vi "CCD-2D-RTmode.vi"() -> ()   [LabVIEW 2021]
uses:
  Globals and TypeDefs/gDetector.vi
panel:
  out "Processing":u32
  out "Read":u32
  out "RQS":u32
  out "Start":u32
  in  "stop":bool
  out "Plot":i32[](graph)
  in  "Shutter Enabled":bool=TRUE
  out "\"ST\" status":bool[](array[boolean])
  in  "Exposuretime (s)":dbl=0.5 format="%.2f"
  in  "CCD GPIB Address":u16=1
  out "error out":errorcluster
  out "The Data":i32[][](array[numeric])=[[1198, 1190, 1193, 1194, 1189, 1188, 1196, 1190, 1202, 1191, 1193, 1192, 1199, 1189, 1194, 1189, 1197, 1191, 1187, 1192, 1195, 1189, 1195, 1191, 1199, 1194, 1192, 1191, 1193, 1197, 1193, 1193, 1194, 1200, 1191, 1190, 1187, 1195, 1189, 1188, 1191, 1194, 1187, 1192, 1198, 1193, 1190, 1192, 1190, 1193, 1191, 1190, 1191, 1189, 1192, 1194, 1190, 1193, 1193, 1191, 1194, 1182, 1190, 1188, 1199, 1192, 1196, 1195, 1186, 1189, 1188, 1185, 1194, 1187, 1193, 1194, 1190, 1189, 1189, 1187, 1196, 1195, 1191, 1197, 1192, 1200, 1187, 1194, 1189, 1193, 1195, 1196, 1186, 1192, 1190, 1194, 1194, 1190, 1191, 1193, 1197, 1197, 1185, 1199, 1190, 1195, 1196, 1184, 1193, 1193, 1193, 1191, 1189, 1190, 1199, 1193, 1191, 1194, 1191, 1192, 1186, 1190, 1194, 1189, 1194, 1190, 1191, 1192, 1192, 1196, 1192, 1192, 1189, 1193, 1198, 1186, 1191, 1193, 1187, 1194, 1190, 1190, 1191, 1189, 1194, 1195, 1189, 1192, 1185, 1193, 1192, 1192, 1189, 1191, 1191, 1190, 1196, 1194, 1193, 1191, 1189, 1191, 1196, 1192, 1192, 1189, 1196, 1191, 1193, 1192, 1188, 1190, 1194, 1192, 1185, 1191, 1194, 1191, 1189, 1195, 1192, 1196, 1190, 1193, 1191, 1189, 1194, 1195, 1191, 1187, 1190, 1196, 1196, 1192, 1197, 1191, 1189, 1192, 1192, 1200, 1192, 1193, 1190, 1192, 1187, 1198, 1186, 1196, 1201, 1199, 1200, 1191, 1196, 1200, 1192, 1191, 1193, 1185, 1192, 1194, 1186, 1190, 1188, 1189, 1201, 1197, 1191, 1194, 1193, 1194, 1195, 1198, 1200, 1192, 1192, 1193, 1193, 1195, 1187, 1193, 1192, 1187, 1189, 1186, 1191, 1197, 1191, 1200, 1194, 1192, 1187, 1196, 1191, 1191, 1196, 1187, 1190, 1193, 1189, 1193, 1190, 1188, 1188, 1190, 1197, 1188, 1191, 1195, 1188, 1191, 1188, 1194, 1193, 1187, 1200, 1192, 1197, 1190, 1196, 1200, 1191, 1189, 1193, 1189, 1186, 1196, 1185, 1198, 1195, 1186, 1191, 1197, 1191, 1193, 1195, 1193, 1191, 1198, 1189, 1183, 1200, 1197, 1192, 1192, 1192, 1196, 1191, 1190, 1194, 1188, 1198, 1193, 1195, 1190, 1187, 1192, 1191, 1195, 1188, 1190, 1191, 1187, 1189, 1185, 1189, 1196, 1198, 1191, 1190, 1196, 1197, 1193, 1187, 1186, 1195, 1191, 1193, 1192, 1196, 1190, 1192, 1192, 1192, 1190, 1195, 1192, 1191, 1193, 1197, 1184, 1190, 1188, 1192, 1194, 1190, 1193, 1195, 1195, 1194, 1189, 1193, 1191, 1194, 1186, 1189, 1192, 1191, 1182, 1190, 1197, 1194, 1188, 1193, 1191, 1186, 1194, 1197, 1193, 1191, 1187, 1194, 1194, 1191, 1189, 1195, 1194, 1189, 1196, 1187, 1186, 1192, 1194, 1196, 1191, 1193, 1191, 1188, 1190, 1199, 1198, 1196, 1196, 1190, 1194, 1191, 1194, 1187, 1195, 1190, 1194, 1196, 1194, 1189, 1193, 1189, 1194, 1189, 1195, 1192, 1194, 1193, 1191, 1197, 1187, 1189, 1189, 1188, 1197, 1192, 1189, 1193, 1194, 1183, 1202, 1187, 1192, 1184, 1188, 1186, 1193, 1189, 1195, 1189, 1193, 1197, 1189, 1194, 1191, 1194, 1192, 1191, 1191, 1196, 1194, 1190, 1193, 1192, 1195, 1197, 1198, 1193, 1202, 1196, 1194, 1194, 1190, 1193, 1190, 1195, 1192, 1187, 1194, 1197, 1190, 1194, 1189, 1198, 1192, 1191, 1192, 1192, 1191, 1191, 1193, 1191, 1191, 1198, 1186, 1192, 1185, 1185, 1188, 1194, 1196, 1194, 1195, 1190, 1194, 1191, 1190, 1195, 1191, 1191, 1195, 1192, 1194, 1201, 1187, 1191, 1195, 1187, 1192, 1192, 1193, 1200, 1188, 1189, 1189, 1197, 1189, 1188, 1197, 1195, 1191, 1189, 1190, 1195, 1189, 1191, 1194, 1186, 1192, 1190, 1191, 1188, 1195, 1192, 1191, 1191, 1199, 1190, 1190, 1190, 1192, 1187, 1193, 1197, 1197, 1186, 1193, 1189, 1192, 1197, 1184, 1187, 1188, 1192, 1192, 1192, 1189, 1192, 1190, 1194, 1191, 1186, 1196, 1194, 1189, 1193, 1191, 1186, 1189, 1193, 1195, 1196, 1197, 1199, 1194, 1190, 1193, 1194, 1190, 1198, 1196, 1194, 1195, 1194, 1184, 1188, 1195, 1197, 1190, 1194, 1190, 1191, 1195, 1198, 1188, 1193, 1194, 1195, 1198, 1195, 1191, 1197, 1192, 1198, 1190, 1196, 1191, 1194, 1188, 1189, 1198, 1192, 1198, 1195, 1185, 1191, 1193, 1192, 1197, 1195, 1195, 1195, 1193, 1190, 1190, 1190, 1198, 1195, 1191, 1194, 1190, 1190, 1194, 1194, 1195, 1192, 1190, 1194, 1195, 1192, 1192, 1194, 1189, 1192, 1193, 1188, 1194, 1195, 1196, 1193, 1192, 1201, 1191, 1198, 1197, 1191, 1192, 1191, 1194, 1193, 1188, 1192, 1189, 1183, 1189, 1190, 1192, 1189, 1196, 1193, 1197, 1185, 1193, 1189, 1191, 1196, 1195, 1193, 1193, 1191, 1189, 1193, 1192, 1192, 1192, 1190, 1191, 1193, 1193, 1197, 1195, 1189, 1193, 1188, 1194, 1197, 1194, 1195, 1196, 1190, 1194, 1188, 1197, 1195, 1191, 1195, 1192, 1194, 1188, 1190, 1197, 1197, 1191, 1187, 1197, 1191, 1193, 1188, 1191, 1194, 1193, 1195, 1192, 1195, 1189, 1193, 1193, 1195, 1190, 1192, 1196, 1188, 1187, 1193, 1192, 1192, 1194, 1185, 1199, 1190, 1193, 1191, 1198, 1189, 1190, 1191, 1190, 1193, 1195, 1186, 1190, 1193, 1191, 1189, 1197, 1193, 1198, 1190, 1192, 1193, 1191, 1196, 1193, 1196, 1190, 1190, 1198, 1192, 1199, 1198, 1190, 1191, 1191, 1196, 1190, 1196, 1195, 1191, 1196, 1195, 1193, 1190, 1190, 1195, 1193, 1187, 1197, 1185, 1191, 1189, 1191, 1193, 1192, 1188, 1196, 1193, 1191, 1193, 1193, 1190, 1192, 1192, 1192, 1195, 1191, 1195, 1189, 1189, 1191, 1191, 1185, 1192, 1191, 1193, 1201, 1199, 1197, 1206, 1201, 1207, 1200, 1198, 1195, 1188, 1194, 1186, 1190, 1197, 1188, 1193, 1196, 1193, 1192, 1192, 1188, 1196, 1186, 1193, 1194, 1188, 1190, 1190, 1192, 1190, 1191, 1191, 1200, 1192, 1199, 1193, 1190, 1190, 1199, 1187, 1193, 1190, 1188, 1194, 1194, 1196, 1194, 1195, 1190, 1187, 1187, 1196, 1193, 1199, 1190, 1193, 1193, 1191, 1198, 1192, 1193, 1192, 1193, 1189, 1189, 1197, 1189, 1194, 1193, 1192, 1185, 1198, 1193, 1189, 1192, 1193, 1196, 1190, 1195, 1189, 1196, 1198, 1190, 1191, 1193, 1186, 1189, 1195, 1188, 1197, 1188, 1191, 1185, 1190, 1193, 1188, 1198, 1192, 1193, 1194, 1194, 1189, 1184, 1193, 1199, 1193, 1192, 1193, 1190, 1196, 1191, 1192, 1189, 1194, 1188, 1189, 1190, 1190, 1192, 1195, 1188, 1190, 1192, 1189, 1197, 1192, 1194, 1187, 1196, 1192, 1194, 1185, 1187, 1187, 1191, 1195, 1190, 1186, 1183, 1194, 1194, 1192, 1192, 1188, 1193, 1195, 1189, 1190, 1191, 1192, 1196, 1186, 1195, 1191, 1185, 1191, 1187, 1190, 1188, 1189, 1187, 1196, 1191, 1190, 1191, 1190, 1196, 1195, 1186, 1187, 1187, 1188, 1194, 1192, 1192, 1192, 1189, 1192, 1191, 1188, 1188, 1187, 1187, 1190, 1186, 1191, 1195, 1192, 1196, 1193, 1192, 1191, 1189, 1187, 1193, 1188, 1189, 1194, 1191, 1185, 1193, 1191, 1196, 1196, 1199, 1195, 1211]]
  out "Setup String":string="ldu,0,256,16;sdu,0,1024,1024;cl0;omrm;sron"
  out "Array Length":i32=1024
  out "sd":i32=1024
  out "ld":i32=16
  out "InitialArray Length":i32=16384
  out "PixelOverflow":bool
  out "RQS  poll response":i16
  out "read status":bool[](array[boolean])
  out "#PixelOverflow":u32
  out "Data Dimensions":i32[](array[numeric])
  out "Intensity Graph":i32[][](graph)
  # "Wait time (ms)"
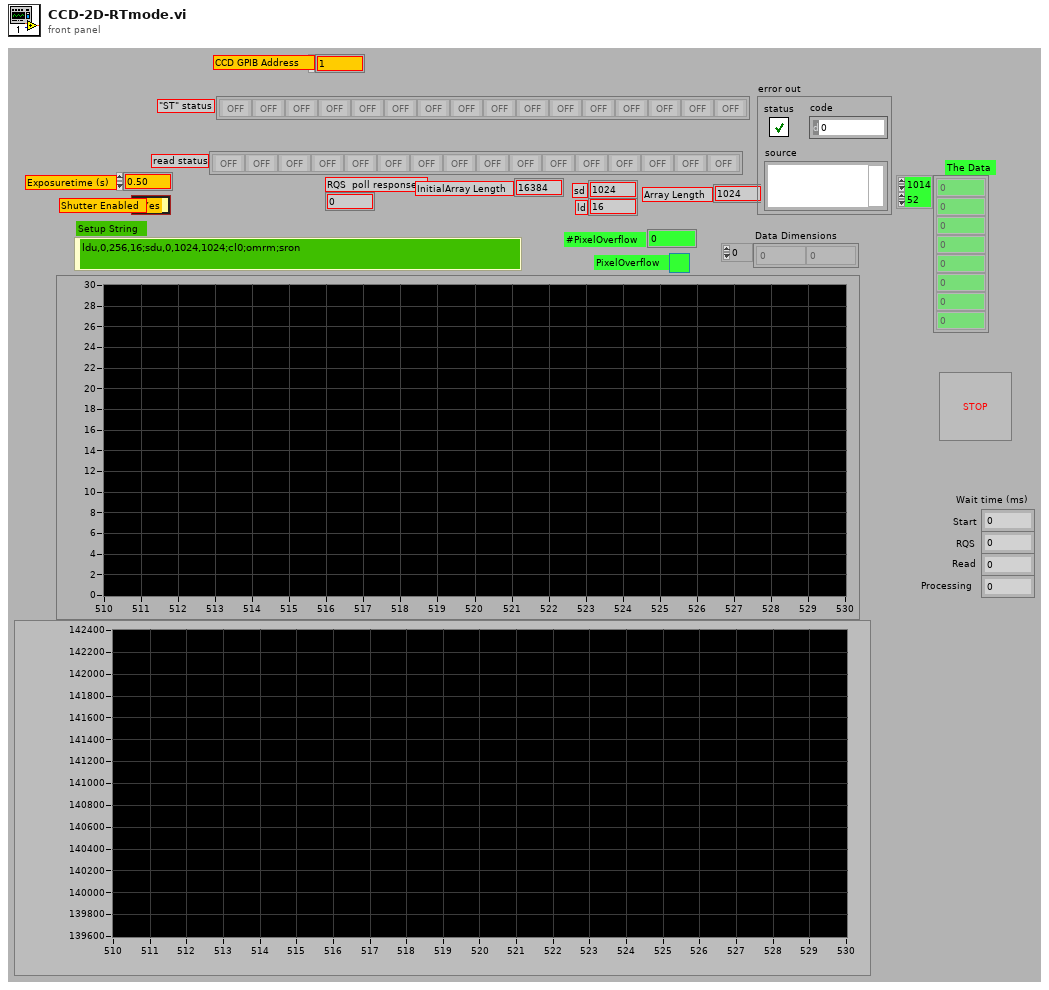
[diagram p1: front panel]
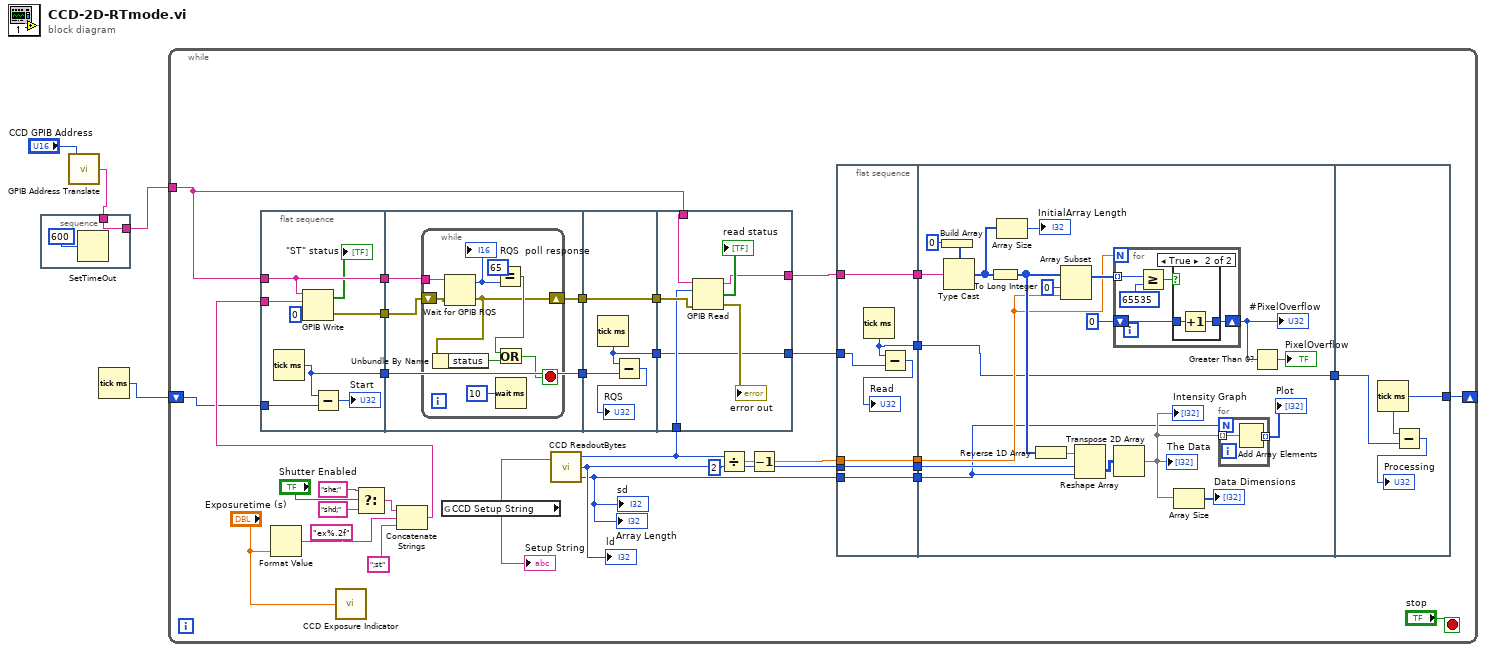
[diagram p0: block diagram]
diagram:
  n1 = call "GPIB Address Translate.vi"("GPIB Address"="CCD GPIB Address") -> ("GPIB Address String"=w3:string)
  n2 = stacked-sequence {
    tunnel: [w5] -> w2
    tunnel: w3 -> [w5]
    frame #0 {
      n3 = SetTimeOut(1:600) -> ()  [unwired: 1 out]
    }
  }
  n4 = Tick Count (ms)() -> (millisecond timer value=w1:u32)
  n5 = while {
    tunnel: w2 -> [w18]
    shift-right: [w15] -> _
    shift-left: w1 -> [w16]
    stop <- "stop" stop-if-true
    n6 = flat-sequence {
      tunnel: w18 -> [w87]
      tunnel: [w87] -> w26
      tunnel: w24 -> [w88]
      tunnel: [w85] -> w23
      tunnel: [w84] -> w21
      tunnel: w16 -> [w83]
      tunnel: w26 -> [w92]
      tunnel: [w93] -> w25
      tunnel: w23 -> [w91]
      tunnel: [w90] -> w22
      tunnel: w21 -> [w90]
      tunnel: w25 -> [w106]
      tunnel: w22 -> [w105]
      tunnel: [w106] -> w20
      tunnel: [w103] -> w9
      tunnel: w20 -> [w112]
      tunnel: w19 -> [w110]
      tunnel: w18 -> [w109]
      tunnel: [w108] -> w17
      tunnel: [w107] -> w10
      tunnel: w9 -> [w107]
      frame #0 {
        n7 = Tick Count (ms)() -> (millisecond timer value=w84:u32)
        n8 = GPIB Write(0:w87, 1:w88, 2:i16 0 ("mode (0)")) -> (5:→"\"ST\" status":bool[], 6:w85:errorcluster)  [unwired: 2 in]
        n9 = Subtract(x=w84, y=w83) -> (x-y=→"Start":u32)
      }
      frame #1 {
        n10 = while {
          tunnel: w92 -> [w102]
          shift-right: [w98] -> w93
          shift-left: w91 -> [w101]
          stop <- w99 stop-if-true
          n11 = Wait for GPIB RQS(2:w101, 4:w102) -> (0:w98:errorcluster, 1:w96:i16)  [unwired: 1 in]
          "RQS  poll response" <- w96
          n12 = Unbundle By Name(w98) -> ("status"=w97:bool)
          n13 = Equal?(x=i16 65 ("y"), y=w96) -> (x = y?=w100:bool)
          n14 = Or(x=w100, y=w97) -> (x .or. y?=w99:bool)
          n15 = Wait (ms)(milliseconds to wait=u32 10) -> ()  [unwired: 1 out]
        }
      }
      frame #2 {
        n16 = Tick Count (ms)() -> (millisecond timer value=w103:u32)
        n17 = Subtract(x=w103, y=w105) -> (x-y=→"RQS":u32)
      }
      frame #3 {
        n18 = GPIB Read(0:w109, 1:w110, 3:w112) -> (5:w108:string, 6:→"read status":bool[], 7:→"error out":errorcluster)  [unwired: 2 in]
      }
    }
    n19 = Format Value(format string="ex%.2f", value (0)="Exposuretime (s)") -> (output string=w32:string)  [unwired: 1 in]
    n20 = call "CCD Exposure Indicator.vi"("ExpTime"="Exposuretime (s)") -> ()  [unwired: 4 in]
    n21 = Select(t="she;", s="Shutter Enabled", f="shd;") -> (s? t:f=w33:string)
    n22 = Concatenate Strings(w33, w32, ";st") -> (w24:string)
    n23 = global read "gDetector.vi" "CCD Setup String"() -> (w39:string)
    "Setup String" <- w39
    n24 = call "CCD ReadoutBytes.vi"("CCD Setup String"=w39) -> ("Bytes for Readout"=w19:i32, "LD Bytes"=w30:i32, "SD Bytes"=w29:i32)  [unwired: 1 in, 1 out]
    "Array Length" <- w29
    "sd" <- w29
    "ld" <- w30
    n25 = Divide(x=w19, y=2) -> (x/y=w40:dbl)
    n26 = Decrement(x=w40) -> (x-1=w38:dbl)
    n27 = flat-sequence {
      tunnel: w17 -> [w45]
      tunnel: w29 -> [w46]
      tunnel: w30 -> [w47]
      tunnel: w38 -> [w48]
      tunnel: [w48] -> w14
      tunnel: [w47] -> w13
      tunnel: [w46] -> w12
      tunnel: [w45] -> w11
      tunnel: w10 -> [w43]
      tunnel: [w42] -> w7
      tunnel: w14 -> [w55]
      tunnel: w13 -> [w53]
      tunnel: w12 -> [w51]
      tunnel: w11 -> [w50]
      tunnel: [w49] -> w8
      tunnel: w7 -> [w49]
      tunnel: [w80] -> w15
      tunnel: w8 -> [w79]
      frame #0 {
        n28 = Tick Count (ms)() -> (millisecond timer value=w42:u32)
        n29 = Subtract(x=w42, y=w43) -> (x-y=→"Read":u32)
      }
      frame #1 {
        n30 = Build Array(u16 0) -> (w66:u16[])
        n31 = Type Cast(type=w66, x=w50) -> (*(type *) &x=w68:u16[])
        n32 = To Long Integer(number=w68) -> (32bit integer=w61:i32[])
        n33 = Array Size(array=w68) -> (size(s)=→"InitialArray Length":i32)
        n34 = Reverse 1D Array(array=w61) -> (reversed array=w63:i32[])
        n35 = Array Subset(array=w61, index=0, length=w55) -> (w60:i32[])
        n36 = Reshape Array(w63, w53, w51) -> (w64:i32[][])
        n37 = for {
          N: w55 -> [_]
          tunnel: w60 -> [w75] mode=indexing
          shift-right: [w73] -> w58
          shift-left: u32 0 -> [w72]
          n38 = Greater Or Equal?(x=w75, y=65535) -> (x >= y?=w74:bool)
          n39 = case shown="True" w74 {
            tunnel: [w76 w78] -> w73
            tunnel: w72 -> [w76 w77]
            frame False {
            }
            frame True {
              n40 = Increment(x=w77) -> (x+1=w78:u32)
            }
          }
        }
        "#PixelOverflow" <- w58
        n41 = Transpose 2D Array(2D array=w64) -> (transposed array=w54:i32[][])
        "The Data" <- w54
        "Intensity Graph" <- w54
        n42 = Array Size(array=w54) -> (size(s)=→"Data Dimensions":i32[])
        n43 = for {
          N: w51 -> [_]
          tunnel: [w70] -> w52 mode=indexing
          tunnel: w54 -> [w69] mode=indexing
          n44 = Add Array Elements(numeric array=w69) -> (sum=w70:i32)
        }
        "Plot" <- w52
        n45 = Greater Than 0?(x=w58) -> (x > 0?=→"PixelOverflow":bool)
      }
      frame #2 {
        n46 = Tick Count (ms)() -> (millisecond timer value=w80:u32)
        n47 = Subtract(x=w80, y=w79) -> (x-y=→"Processing":u32)
      }
    }
  }
